vi "1_10_filter (delete).vi"(0 "input":dbl, 1 "reset":bool) -> (4 "output":dbl)   [LabVIEW 2019]
doc: "Applies a fifth-order low-pass integer FIR filter to the input data. The filter cut-off frequency is 1/10 of the sample frequency of the <B>input</B>. Use the Discrete Control Filter VI to filter measured values, such as the process variable, in control applications. The data type you wire to <B>input</B> determines the <B>output</B> data type."
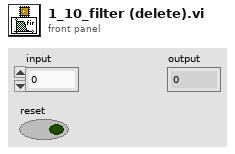
[diagram p1: front panel]
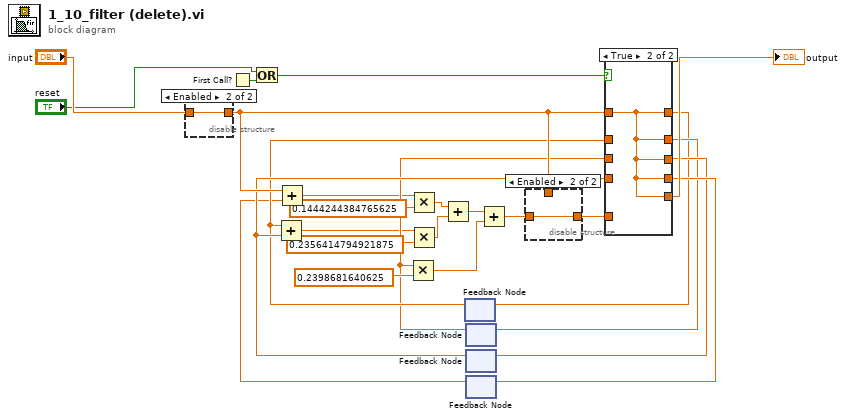
[diagram p0: block diagram]
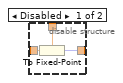
[diagram p2: hidden frame]
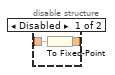
[diagram p3: hidden frame]
diagram:
  n1 = disable-structure shown="Enabled" {
    disable-tunnel: "input" -> [w27 w28]
    disable-tunnel: [w26 w28] -> w19
    frame Disabled {
      n2 = To Fixed-Point(number=w27) -> (fixed-point=w26:fxp<+/-,21,-4>)  [unwired: 1 in]
    }
    frame Enabled {
    }
  }
  n3 = First Call?() -> (First Call?: T/F=w11:bool)
  n4 = Or(x="reset", y=w11) -> (x .or. y?=w10:bool)
  n5 = feedback #1() -> (w13:dbl)  [unwired: 1 in]
  n6 = feedback #2() -> (w9:dbl)  [unwired: 1 in]
  n7 = Multiply(x=w9, y=0.2398681640625) -> (x*y=w17:dbl)
  n8 = feedback #3() -> (w14:dbl)  [unwired: 1 in]
  n9 = Add(x=w13, y=w14) -> (x+y=w7:dbl)
  n10 = Multiply(x=w7, y=0.2356414794921875) -> (x*y=w8:dbl)
  n11 = feedback #4() -> (w12:dbl)  [unwired: 1 in]
  n12 = Add(x=w19, y=w12) -> (x+y=w5:dbl)
  n13 = Multiply(x=w5, y=0.1444244384765625) -> (x*y=w6:dbl)
  n14 = Add(x=w6, y=w8) -> (x+y=w16:dbl)
  n15 = Add(x=w16, y=w17) -> (x+y=w18:dbl)
  n16 = disable-structure shown="Enabled" {
    disable-tunnel: w19 -> [w31 _]
    disable-tunnel: w18 -> [w30 w32]
    disable-tunnel: [w29 w32] -> w15
    frame Disabled {
      n17 = To Fixed-Point(fixed-point type=w31, number=w30) -> (fixed-point=w29:fxp<+/-,21,-4>)
    }
    frame Enabled {
    }
  }
  n18 = case shown="True" w10 {
    tunnel: [w37 w38] -> w1
    tunnel: w19 -> [w37 w38]
    tunnel: [w36 w38] -> w2
    tunnel: [w35 w38] -> w3
    tunnel: [w34 w38] -> w4
    tunnel: w9 -> [w35 _]
    tunnel: w14 -> [w34 _]
    tunnel: w13 -> [w36 _]
    tunnel: w15 -> [w33 _]
    tunnel: [w33 w38] -> w23
    frame False {
    }
    frame True {
    }
  }
  "output" <- w23
  n19 = feedback-in #1(w1) -> ()
  n20 = feedback-in #2(w2) -> ()
  n21 = feedback-in #3(w3) -> ()
  n22 = feedback-in #4(w4) -> ()
